vi "Get Object Pointer.vi"(11 "Event in":refnum<class "Event.lvclass">) -> (1 "Object Pointer":i64, 2 "Assigned object pointer?":bool, 3 "Event out":refnum<class "Event.lvclass">)   [LabVIEW 2013, in "MDSplus.lvlib" / "Event.lvclass"]
uses:
  <vilib>/MDSplus/Classes/Event_Class/Event.lvclass
  <vilib>/MDSplus/Classes/Event_Class/Event.lvclass/Event.ctl
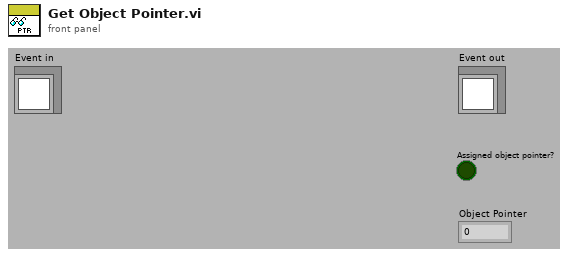
[diagram p1: front panel]
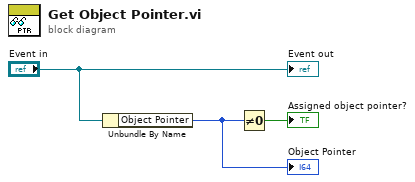
[diagram p0: block diagram]
diagram:
  n1 = Unbundle By Name("Event in") -> ("Object Pointer"=w1:i64)
  "Object Pointer" <- w1
  n2 = Not Equal To 0?(x=w1) -> (x != 0?=→"Assigned object pointer?":bool)
  "Event out" <- "Event in"
